vi "Self-Balancing-LINX-Code.vi"() -> ()   [LabVIEW 2021]
uses:
  <vilib>/MakerHub/LINX/Public/Sensors/Accelerometer/MPU60X0/DeviceAddresses.ctl
  <vilib>/MakerHub/LINX/Public/Sensors/Accelerometer/MPU60X0/GyroFullScaleRanges.ctl
  <vilib>/MakerHub/LINX/Public/Utilities/Open Serial.vi
  <vilib>/MakerHub/LINX/LMH-LINX.lvlib
  <vilib>/MakerHub/LINX/Public/Sensors/Accelerometer/MPU60X0/MPU60X0.lvlib
panel:
  in  "Gyro_Weight":dbl=0.99 format="%#_13g"
  in  "Accel Weight":dbl=0.01 format="%#_13g"
  in  "Ki":dbl=0.01
  in  "milliseconds to wait":ext=1.0
  out "Gyro Angle Chart":ext(graph)=0.15136363636363636363
  in  "Kd":dbl=0.03
  out "Accelerometer Angle Chart":dbl(graph)
  out "Saturated PD":dbl=47.931426005026836
  in  "Scale_Offset":ext=2.2
  in  "Offset":i16=333
  out "Motor PWM":dbl=47.931426005026836
  out "PID":dbl=47.931426005026836
  in  "Kp":dbl=30.0
  out "Filtered Angle Chart":ext(graph)=0.14984999999999999865
  # "PD Control"
  # "Gyro Offset"
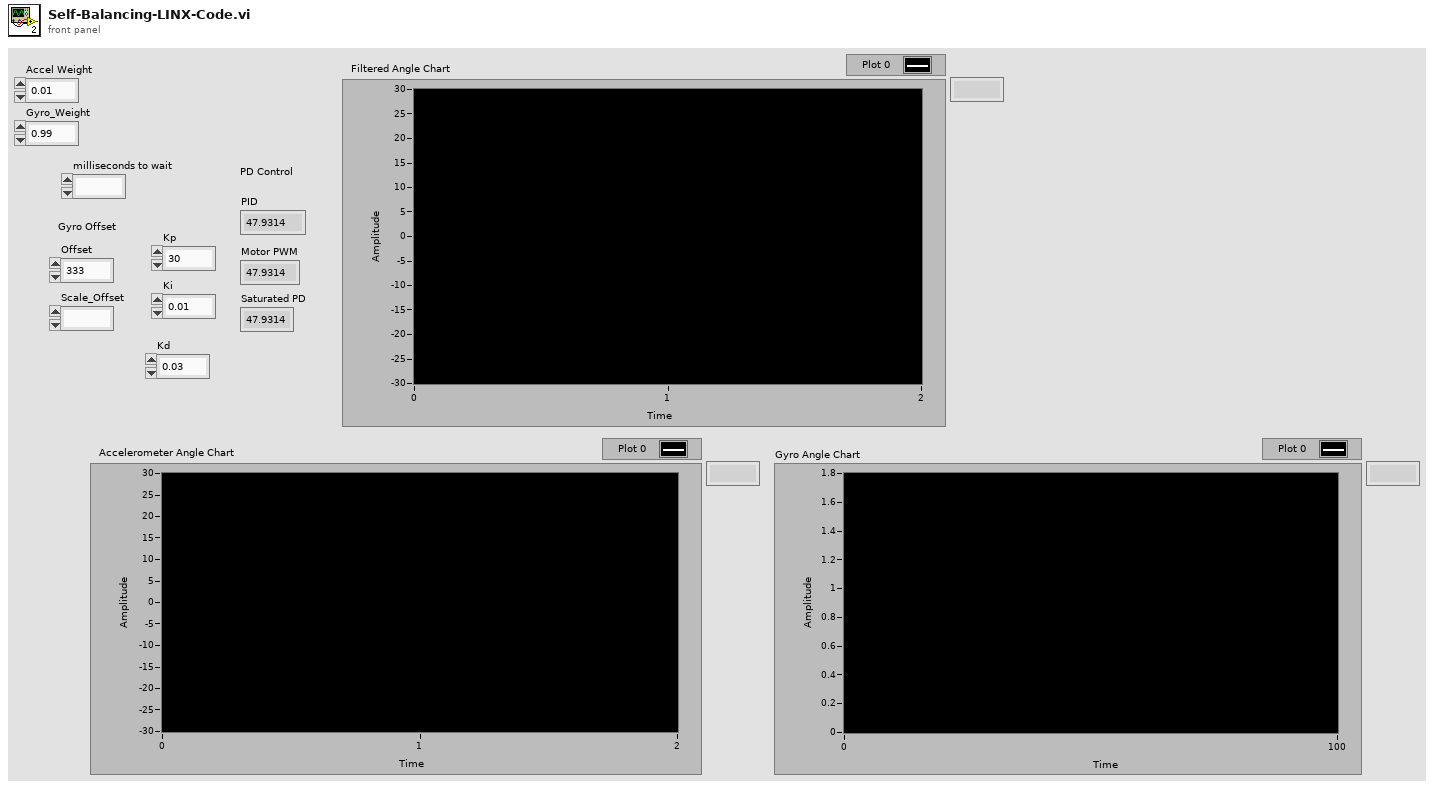
[diagram p1: front panel]
types:
  T1 = typedef "LMH-LINX.lvlib/MPU60X0.lvlib/GyroFullScaleRanges.ctl" = enum8{"±250 °/s", "±500 °/s", "±1000 °/s", "±2000 °/s"}
  T2 = typedef "LMH-LINX.lvlib/MPU60X0.lvlib/DeviceAddresses.ctl" = enum16{"0x68", "0x69"}
  T3 = typedef "LMH-LINX.lvlib/LINX Ref.ctl" = cluster{"IO":T4, "Interface":T5, "LINX Device Config":T6}
  T4 = typedef "LMH-LINX.lvlib/Platform.ctl" = enum16{"Remote", "Local"}
  T5 = typedef "LMH-LINX.lvlib/Interface.ctl" = enum16{"Serial", "TCP"}
  T6 = typedef "LMH-LINX.lvlib/Device.lvlib/LINX Device Config.ctl" = cluster{"Interface":T5, "COM Port":refnum<visa-resource-name>, "TCP Configuration":T7, "Device Family":u8, "Device ID":u8, "Device Name":string, "TCP Ref":refnum<k5>, "Channels":T8}
  T7 = typedef "LMH-LINX.lvlib/Device.lvlib/TCP Config.ctl" = cluster{"IP Address":string, "Port":u16}
  T8 = typedef "LMH-LINX.lvlib/Channels.ctl" = cluster{"DI":u8[], "DO":u8[], "AI":u8[], "AO":u8[], "PWM":u8[], "QE":u8[], "UART":u8[], "I2C 2":u8[], "SPI":u8[], "CAN":u8[], "Servo":u8[], "AI Ref (V)":dbl, "AI Resolution (Bits)":u8, "AO Ref (V)":dbl, "AO Resolution (Bits)":u8}
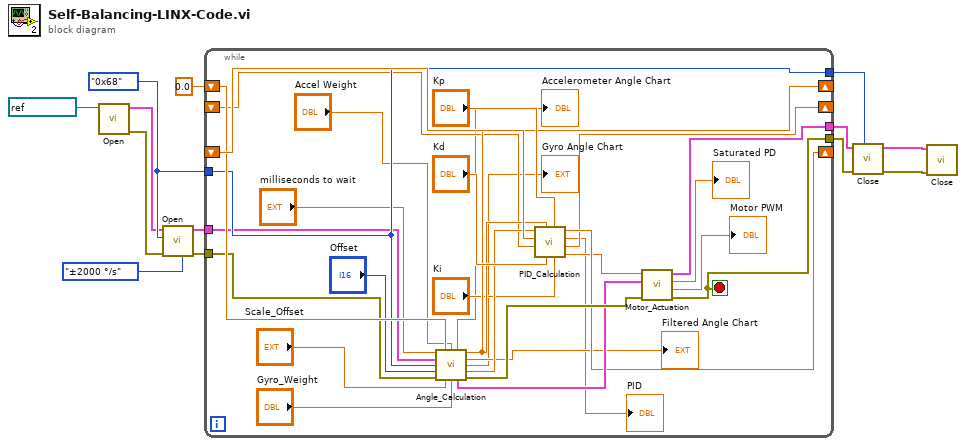
[diagram p0: block diagram]
diagram:
  w13 = DeviceAddresses."0x68" ("I2C Slave Address")
  n1 = call-poly <vilib>:"Open.vi"("Serial Port"=refnum<visa-resource-name> "COM10") -> ("Error Out"=w8:errorcluster, "LINX Resource"=w11:T3)  [unwired: 8 in, 1 out]
  n2 = call <vilib>:"Open.vi"("Gyro Full Scale Range"=GyroFullScaleRanges."±2000 °/s", "Error In"=w8, "I2C Slave Address"=w13, "LINX Resource"=w11) -> ("Error Out"=w9:errorcluster, "LINX Resource"=w10:T3)  [unwired: 6 in]
  n3 = while {
    tunnel: w13 -> [w36]
    tunnel: [w36] -> w3
    tunnel: w10 -> [w35]
    tunnel: [w42] -> w7
    tunnel: [w41] -> w4
    tunnel: w9 -> [w37]
    shift-right: [w24] -> _
    shift-left: _ -> [w39]
    shift-right: [w27] -> _
    shift-left: 0.0 -> [w38]
    shift-right: [w23] -> _
    shift-left: _ -> [w25]
    stop <- w41 stop-if-true
    n4 = call "Angle_Calculation.vi"("milliseconds to wait in"="milliseconds to wait", "Previous Filtered Angle"=w38, "Accel Weight"="Accel Weight", "LINX Resource in"=w35, "I2C Slave Address"=w36, "Offset"="Offset", "error in (no error)"=w37, "Scale_Offset"="Scale_Offset", "Gyro_Weight"="Gyro_Weight") -> ("Accelerometer Angle Chart"=→"Accelerometer Angle Chart":dbl, "Filtered Angle"=w27:ext, "Filtered Angle Chart"=→"Filtered Angle Chart":ext, "Gyro Angle Chart"=→"Gyro Angle Chart":ext, "milliseconds to wait out"=w26:ext, "LINX Resource out"=w33:T3, "error out"=w34:errorcluster)
    n5 = call "PID_Calculation.vi"("Ki"="Ki", "Kp"="Kp", "Kd"="Kd", "Angle"=w27, "sum_[e(t)*dt]"=w25, "e(t-1)"=w39, "milliseconds to wait in"=w26) -> (0:"PID"=w21:ext, "sum_[e(t)*dt] + new_[e(t)*dt]"=w23:ext, 2:"PID"=→"PID":dbl, "e(t)"=w24:ext)  [unwired: 1 in]
    n6 = call "Motor_Actuation.vi"("error in (no error)"=w34, "LINX Resource in"=w33, "PID"=w21) -> ("error out"=w41:errorcluster, "Motor PWM"=→"Motor PWM":dbl, "Saturated PD"=→"Saturated PD":dbl, "LINX Resource"=w42:T3)  [unwired: 5 in]
  }
  n7 = call <vilib>:"Close.vi"("I2C Channel (0)"=w3, "Error In"=w4, "LINX Resource"=w7) -> ("Error Out"=w5:errorcluster, "LINX Resource"=w6:T3)  [unwired: 7 in]
  n8 = call <vilib>:"Close.vi"("Error In"=w5, "LINX Resource"=w6) -> ()  [unwired: 9 in, 1 out]
